vi "FPGA Target Approach RetractionA2copyAidanV2.vi"() -> ()   [LabVIEW 2012]
uses:
  <vilib>/rvi/FXPMathLib/basic elements/FxpIntAccumulator/subVIs/nifxpmath_IntAccumulator_SimConfig.ctl
  <vilib>/rvi/FXPMathLib/basic elements/FxpIntAccumulator/simVIs/DllFxpIntAccumulator_sub.vi
  <vilib>/rvi/Emulation/niFpgaSctlEmulationGetInTimedLoop.vi
  <vilib>/rvi/Emulation/niFpgaSctlEmulationGlobalWrite.vi
  <vilib>/rvi/eio/common/nirviEmuTemplateMethod_errors.vi
  <vilib>/rvi/interface/RandomDataEmulation/nirviRandomDataFPGAFIFO.vi
  <vilib>/rvi/interface/RandomDataEmulation/niFpgaRandomDataHandleErrors.vi
  <vilib>/rvi/FXPMathLib/basic elements/FxpIntAccumulator/XNode/nifxpmath_IntAccumulator.xnode
  <vilib>/eio/EIONode/EIONode.xnode
  <vilib>/rvi/Analysis/measure/butterworth/XNode/niFpgaButterworthFilter.xnode
  <vilib>/rvi/DataTransferAndStorage/Container/XNode/niFpgaContainer.xnode
  <vilib>/rvi/interface/RandomDataEmulation/nirviRandomDataFpgaReadWriteTemplate.vi
panel:
  in  "bounce distance control":i32
  in  "Set \"bounce\" distance or \nretract until":bool
  in  "Stop Fine Retraction\nand start next approach":bool
  out "Connector0/AI2":i16
  out "x*y":fxp<+/-,64,54>
  out "Numeric":i32
  out "initial setup complete":bool
  out "TF Phase":i16
  out "Approaches done and fully retracted":bool
  in  "Current Image":u8
  in  "Total Number of Images":u8
  out "Acoustic Sensor Signal":i16
  out "Step counter":i16
  out "fine indicator":i16
  in  "TF in Air":i32
  in  "Approach Minimum":i32
  in  "Approach Setpoint":i32
  in  "Fast Approach Offset":i32
  out "SummationfA":i32
  in  "Fine Approach Speed":fxp<+,64,38>
  out "SummationfR":i32
  in  "Fine Retraction Speed":fxp<+,64,38>
  out "SummationFA":i32
  out "Test Case Number Indicator":u8 format="%.1f"
  in  "Fast Approach Speed":fxp<+,64,38>
  in  "Approach":bool
  out "SummationFR":i32
  in  "Data Acquisition Rate":i16
  out "Ticks":i16
  out "Acoustic Sensor Phase":i16
  out "Tuning Fork Signal":i16
  in  "Fast Retraction Speed":fxp<+,64,38>
  out "Counter Indicator":fxp<+/-,64,32>
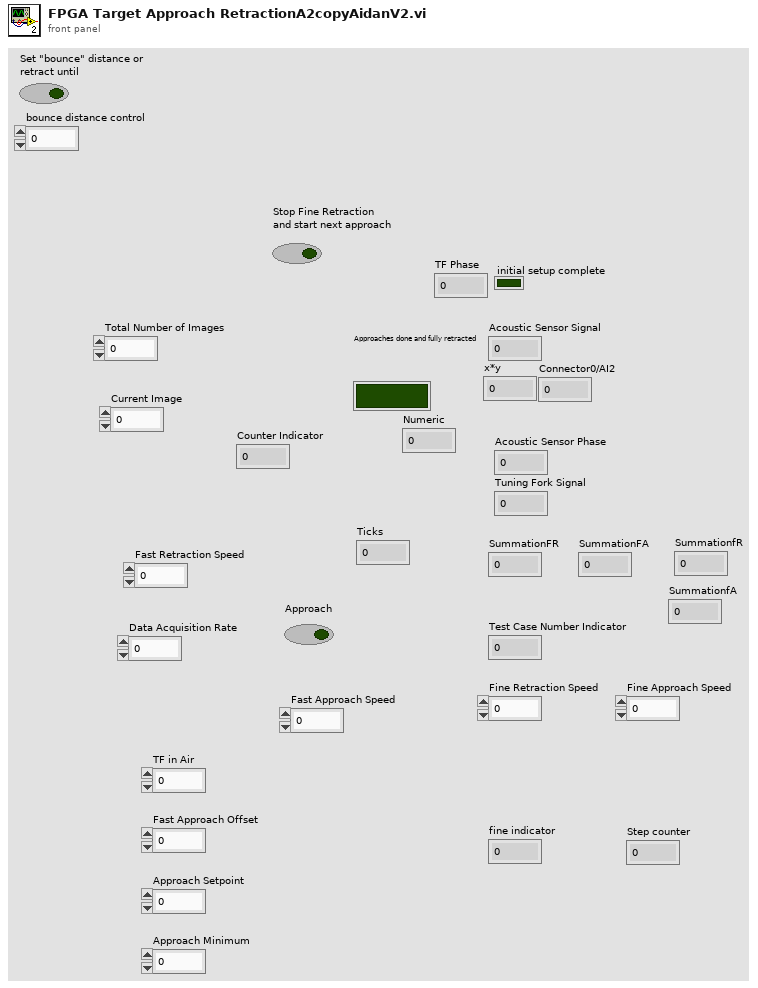
[diagram p1: front panel]
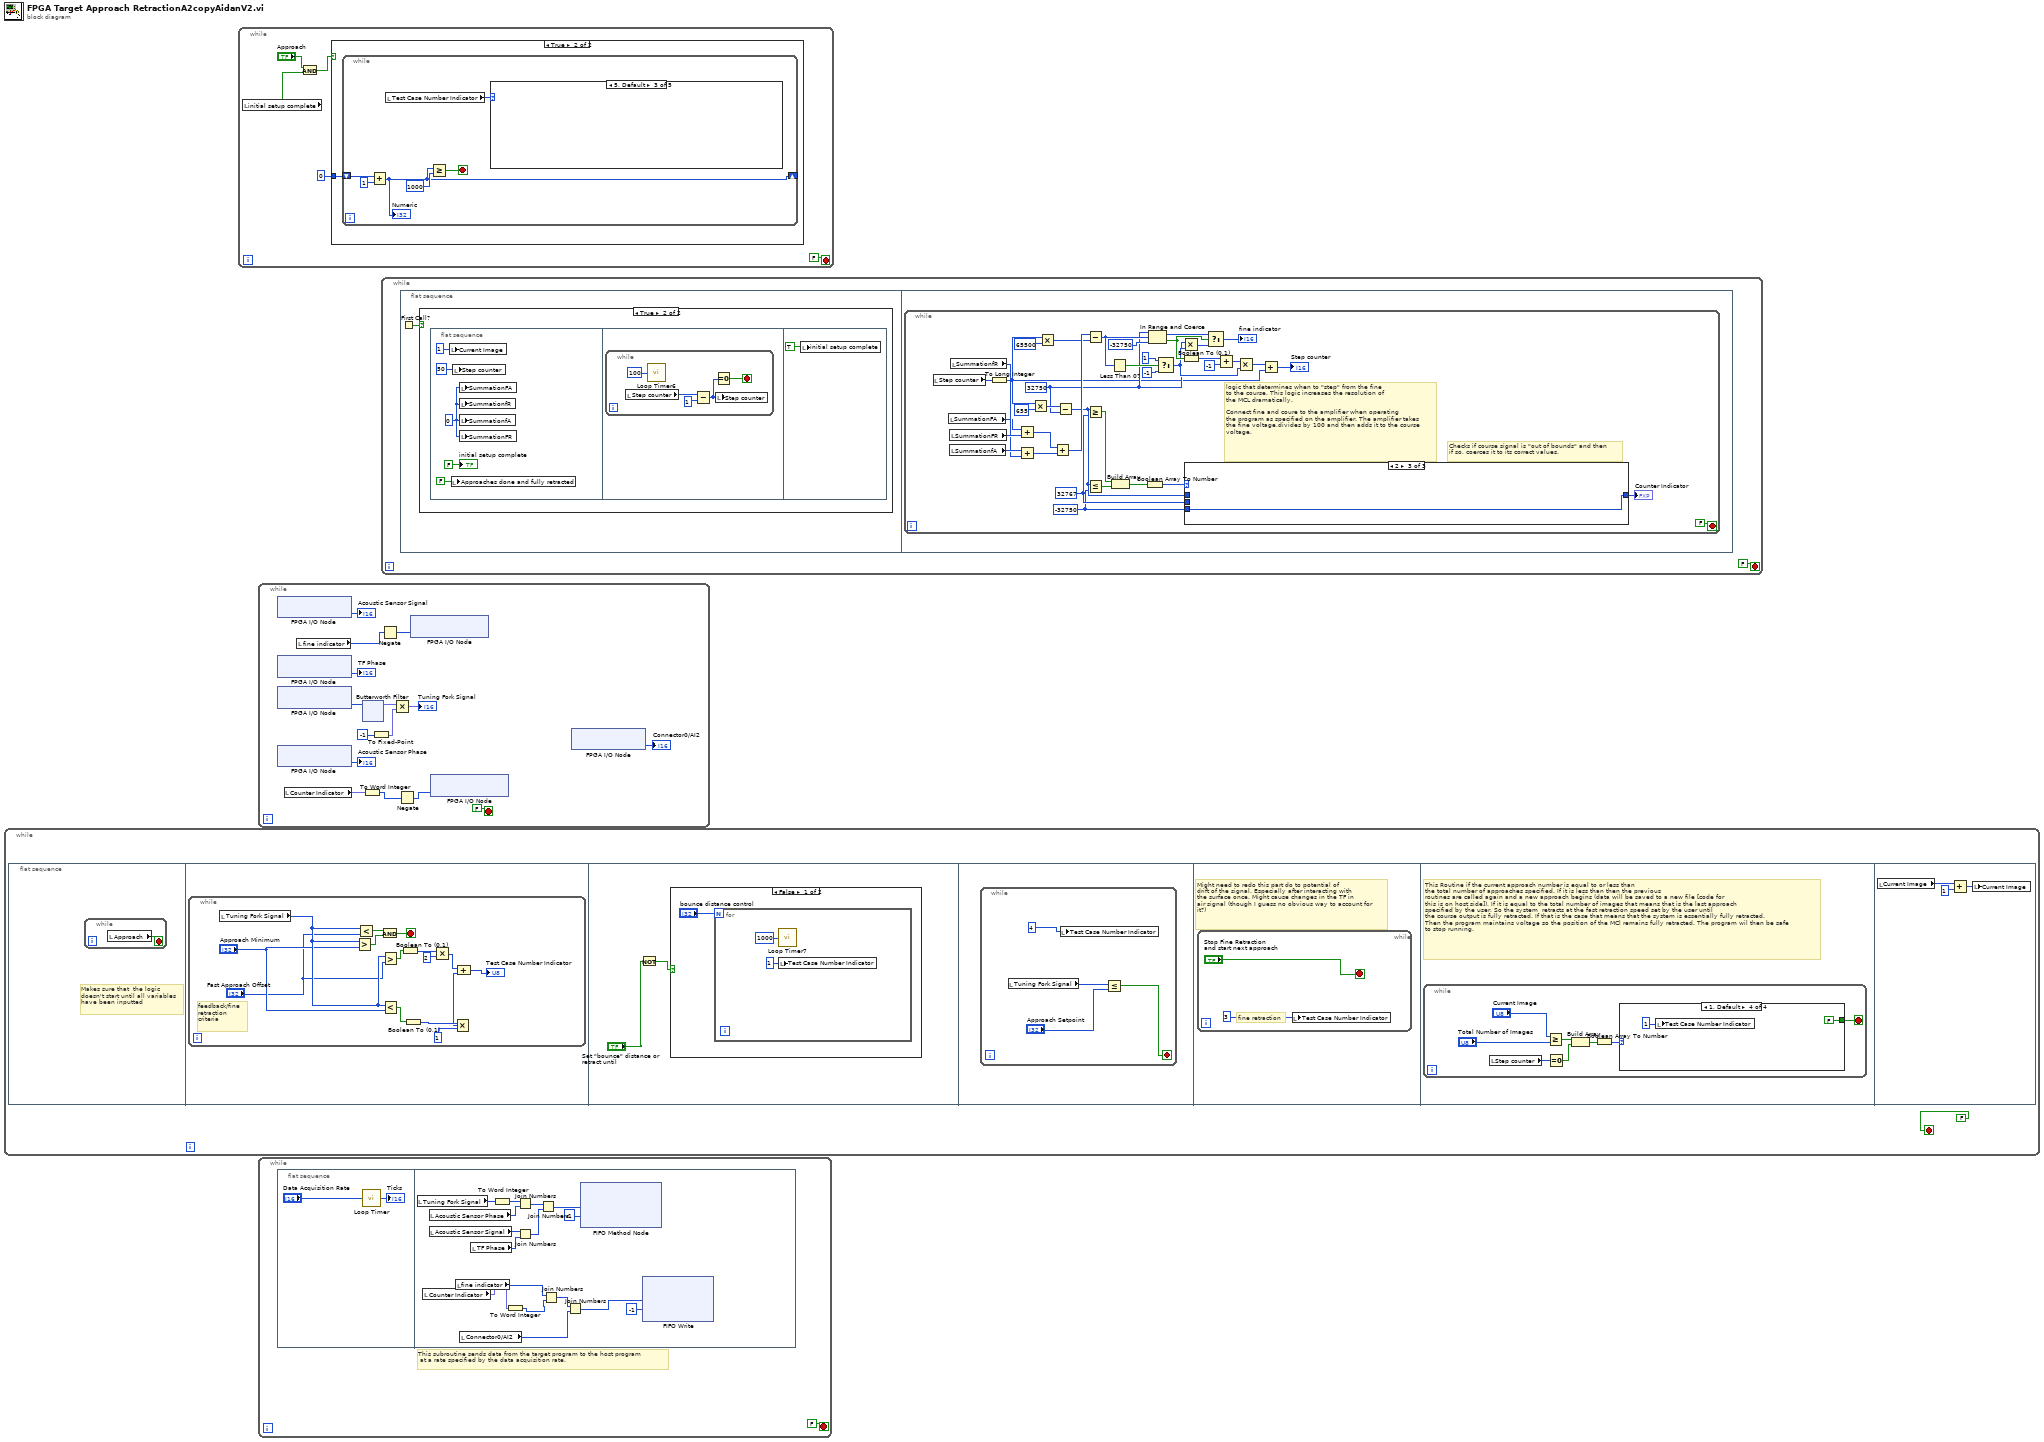
[diagram p0: block diagram]
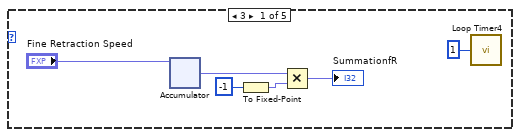
[diagram p3: hidden frame]
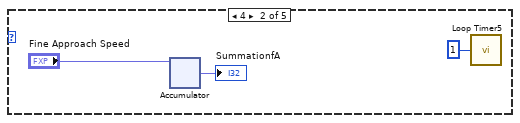
[diagram p4: hidden frame]
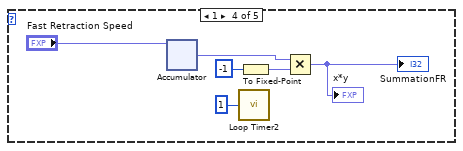
[diagram p5: hidden frame]
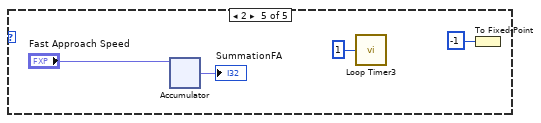
[diagram p6: hidden frame]
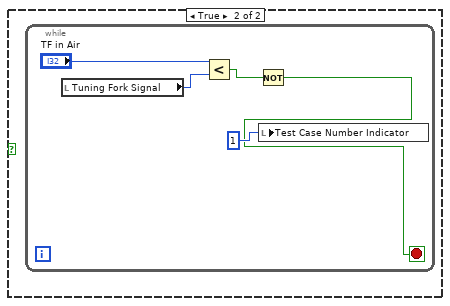
[diagram p10: hidden frame]
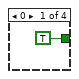
[diagram p11: hidden frame]
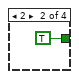
[diagram p12: hidden frame]
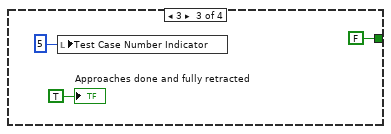
[diagram p13: hidden frame]
diagram:
  n1 = while {
    stop <- FALSE stop-if-true
    n2 = flat-sequence {
      frame #0 {
        # "Makes sure that  the logic  \ndoesn't start until all variables\nhave been inputted"
        n3 = while {
          stop <- w2 stop-if-true
          n4 = local read "Approach"() -> (w2:bool)
        }
      }
      frame #1 {
        n5 = while {
          stop <- w8 stop-if-true
          # "feedback/fine retraction criteria"
          n6 = local read "Tuning Fork Signal"() -> (w11:i16)
          n7 = Greater?(x=w11, y="Approach Minimum") -> (0:w9:bool)
          n8 = Less?(x=w11, y="Fast Approach Offset") -> (x < y?=w10:bool)
          n9 = And(x=w10, y=w9) -> (x .and. y?=w8:bool)
          n10 = Greater?(x=w11, y="Fast Approach Offset") -> (0:w17:bool)
          n11 = Less?(x=w11, y="Approach Minimum") -> (x < y?=w12:bool)
          n12 = Boolean To (0,1)(Boolean=w17) -> (0, 1=w16:i16)
          n13 = Boolean To (0,1)(Boolean=w12) -> (0, 1=w13:i16)
          n14 = Multiply(x=w16, y=i16 2) -> (x*y=w6:i16)
          n15 = Multiply(x=w13, y=i16 1) -> (x*y=w5:i16)
          n16 = Compound Arithmetic op=ADD(w6, w5) -> (→"Test Case Number Indicator":i16)
        }
      }
      frame #2 {
        n17 = Not(x="Set \"bounce\" distance or \nretract until") -> (.not. x?=w18:bool)
        n18 = case shown="False" w18 {
          frame False {
            n19 = for {
              N: "bounce distance control" -> [_]
              n20 = call "Loop Timer7"("Count(mSec)"=u32 1000) -> ()  [unwired: 1 out]
              n21 = local write "Test Case Number Indicator"(u8 1 ("Test Case Number Indicator")) -> ()
            }
          }
          frame True {
            n22 = while {
              stop <- w23 stop-if-true
              n23 = local read "Tuning Fork Signal"() -> (w25:i16)
              n24 = Less?(x="TF in Air", y=w25) -> (x < y?=w24:bool)
              n25 = Not(x=w24) -> (.not. x?=w23:bool)
              n26 = local write "Test Case Number Indicator"(i16 1) -> ()
            }
          }
        }
      }
      frame #3 {
        n27 = while {
          stop <- w28 stop-if-true
          n28 = local read "Tuning Fork Signal"() -> (w29:i16)
          n29 = local write "Test Case Number Indicator"(u8 4 ("Test Case Number Indicator")) -> ()
          n30 = Less Or Equal?(x=w29, y="Approach Setpoint") -> (x <= y?=w28:bool)
        }
      }
      frame #4 {
        # "Might need to redo this part do to potential of\ndrift of the signal. Especially after interacting with \nthe surface once. Might cause changes in the TF in \nair signal (though I guess no obvious way to account for\nit?)"
        n31 = while {
          stop <- "Stop Fine Retraction\nand start next approach" stop-if-true
          # "fine retraction"
          n32 = local write "Test Case Number Indicator"(i16 3) -> ()
        }
      }
      frame #5 {
        # "This Routine if the current approach number is equal to or less than \nthe total number of approaches specified. If it is less than then the previous \nroutines are called again and a new approach begins (data will be saved to a new file [code for \nthis is on host side]). If it is equal to the total number of images that means that is the last approach\nspecified by the user. So the system  retracts at the fast retraction speed set by the user until\nthe course output is fully retracted. If that is the case that means that the system is essentially fully retracted. \nThen the program maintains voltage so the position of the MCl remains fully retracted. The program wil then be safe\nto stop running."
        n33 = while {
          stop <- w34 stop-if-true
          n34 = local read "Step counter"() -> (w39:i16)
          n35 = Greater Or Equal?(x="Current Image", y="Total Number of Images") -> (x >= y?=w38:bool)
          n36 = Equal To 0?(x=w39) -> (x = 0?=w37:bool)
          n37 = Build Array(w38, w37) -> (w36:bool[])
          n38 = Boolean Array To Number(Boolean array=w36) -> (number=w35:u8)
          n39 = case shown="1, Default" w35 {
            tunnel: [TRUE TRUE FALSE FALSE] -> w34
            frame 0 {
            }
            frame 2 {
            }
            frame 3 {
              n40 = local write "Test Case Number Indicator"(i16 5 ("Test Case Number Indicator")) -> ()
              "Approaches done and fully retracted" <- TRUE ("Approaches done and fully retracted")
            }
            frame 1, Default {
              n41 = local write "Test Case Number Indicator"(i16 1) -> ()
            }
          }
        }
      }
      frame #6 {
        n42 = local read "Current Image"() -> (w50:u8)
        n43 = Add(x=w50, y=u8 1) -> (x+y=w49:u8)
        n44 = local write "Current Image"(w49) -> ()
      }
    }
  }
  n45 = while {
    stop <- FALSE stop-if-true
    n46 = local read "initial setup complete"() -> (w53:bool)
    n47 = And(x="Approach", y=w53) -> (x .and. y?=w52:bool)
    n48 = case shown="True" w52 {
      tunnel: i16 0 -> [_ w57]
      frame False {
      }
      frame True {
        n49 = while {
          shift-right: [w58] -> _
          shift-left: w57 -> [w61]
          stop <- w62 stop-if-true
          n50 = Add(x=w61, y=1) -> (x+y=w58:i32)
          "Numeric" <- w58
          n51 = local read "Test Case Number Indicator"() -> (w63:u8)
          n52 = Greater Or Equal?(x=w58, y=1000) -> (x >= y?=w62:bool)
          n53 = case shown="5, Default" w63 {
            frame 3 {
              n54 = xnode "Accumulator"("x"="Fine Retraction Speed") -> ("s"=w64:fxp<+,64,38>)  [unwired: 4 in, 1 out]
              n55 = To Fixed-Point(number=i16 -1) -> (fixed-point=w67:fxp<+/-,16,16>)  [unwired: 1 in]
              n56 = Multiply(x=w64, y=w67) -> (x*y=→"SummationfR":fxp<+/-,64,54>)
              n57 = call "Loop Timer4"("Count(uSec)"=i16 1) -> ()  [unwired: 1 out]
            }
            frame 4 {
              n58 = xnode "Accumulator"("x"="Fine Approach Speed") -> ("s"=→"SummationfA":fxp<+,64,38>)  [unwired: 4 in, 1 out]
              n59 = call "Loop Timer5"("Count(uSec)"=i16 1) -> ()  [unwired: 1 out]
            }
            frame 5, Default {
            }
            frame 1 {
              n60 = xnode "Accumulator"("x"="Fast Retraction Speed") -> ("s"=w130:fxp<+,64,38>)  [unwired: 4 in, 1 out]
              n61 = call "Loop Timer2"("Count(uSec)"=i16 1) -> ()  [unwired: 1 out]
              n62 = To Fixed-Point(number=i16 -1) -> (fixed-point=w128:fxp<+/-,16,16>)  [unwired: 1 in]
              n63 = Multiply(x=w130, y=w128) -> (x*y=→"SummationFR" →"x*y":fxp<+/-,64,54>)
            }
            frame 2 {
              n64 = xnode "Accumulator"("x"="Fast Approach Speed") -> ("s"=→"SummationFA":fxp<+,64,38>)  [unwired: 4 in, 1 out]
              n65 = call "Loop Timer3"("Count(uSec)"=i16 1) -> ()  [unwired: 1 out]
              n66 = To Fixed-Point(number=i16 -1) -> ()  [unwired: 1 in, 1 out]
            }
          }
        }
      }
    }
  }
  n67 = while {
    stop <- FALSE stop-if-true
    n68 = xnode "FPGA I/O Node"() -> ("Connector0/AI5"=→"Acoustic Sensor Signal":i16)  [unwired: 1 in, 1 out]
    n69 = xnode "FPGA I/O Node"() -> ("Connector0/AI4"=→"TF Phase":i16)  [unwired: 1 in, 1 out]
    n70 = xnode "FPGA I/O Node"() -> ("Connector0/AI7"=w200:i16)  [unwired: 1 in, 1 out]
    n71 = xnode "FPGA I/O Node"() -> ("Connector0/AI6"=→"Acoustic Sensor Phase":i16)  [unwired: 1 in, 1 out]
    n72 = local read "Counter Indicator"() -> (w197:fxp<+/-,64,32>)
    n73 = local read "fine indicator"() -> (w193:i16)
    n74 = xnode "Butterworth Filter"("input data"=w200) -> ("output data"=w204:fxp<+/-,20,20>)  [unwired: 2 in]
    n75 = To Word Integer(number=w197) -> (16bit integer=w195:i16)
    n76 = To Fixed-Point(number=i16 -1) -> (fixed-point=w203:fxp<+/-,16,16>)  [unwired: 1 in]
    n77 = Negate(x=w193) -> (-x=w192:i16)
    n78 = Multiply(x=w204, y=w203) -> (x*y=→"Tuning Fork Signal":fxp<+/-,36,36>)
    n79 = Negate(x=w195) -> (-x=w194:i16)
    n80 = xnode "FPGA I/O Node"("Connector0/AO6"=w192) -> ()  [unwired: 1 in, 1 out]
    n81 = xnode "FPGA I/O Node"("Connector0/AO7"=w194) -> ()  [unwired: 1 in, 1 out]
    n82 = xnode "FPGA I/O Node"() -> ("Connector0/AI2"=→"Connector0/AI2":i16)  [unwired: 1 in, 1 out]
  }
  n83 = while {
    stop <- FALSE stop-if-true
    # "This subroutine sends data from the target program to the host program\n at a rate specified by the data acquisition rate."
    n84 = flat-sequence {
      frame #0 {
        n85 = call "Loop Timer"("Count(uSec)"="Data Acquisition Rate") -> ("Tick Count(uSec)"=→"Ticks":u32)
      }
      frame #1 {
        n86 = local read "Tuning Fork Signal"() -> (w231:i16)
        n87 = local read "Counter Indicator"() -> (w222:fxp<+/-,64,32>)
        n88 = local read "Acoustic Sensor Phase"() -> (w229:i16)
        n89 = local read "Acoustic Sensor Signal"() -> (w225:i16)
        n90 = local read "fine indicator"() -> (w218:i16)
        n91 = local read "Connector0/AI2"() -> (w216:i16)
        n92 = local read "TF Phase"() -> (w224:i16)
        n93 = To Word Integer(number=w231) -> (16bit integer=w228:i16)
        n94 = To Word Integer(number=w222) -> (16bit integer=w219:i16)
        n95 = Join Numbers(hi=w228, lo=w229) -> ((hi.lo)=w227:u32)
        n96 = Join Numbers(hi=w225, lo=w224) -> ((hi.lo)=w223:u32)
        n97 = Join Numbers(hi=w227, lo=w223) -> ((hi.lo)=w230:u64)
        n98 = Join Numbers(hi=w218, lo=w219) -> ((hi.lo)=w217:u32)
        n99 = Join Numbers(hi=w217, lo=w216) -> ((hi.lo)=w221:u64)
        n100 = xnode ("FIFO Method Node")("Element"=w230, "Timeout"=i16 -1) -> ()  [unwired: 1 in, 2 out]
        n101 = xnode "FIFO Write"("Element"=w221, "Timeout"=-1) -> ()  [unwired: 1 in, 2 out]
      }
    }
  }
  n102 = while {
    stop <- FALSE stop-if-true
    n103 = flat-sequence {
      frame #0 {
        n104 = First Call?() -> (First Call?: T/F=w233:bool)
        n105 = case shown="True" w233 {
          frame False {
          }
          frame True {
            n106 = flat-sequence {
              frame #0 {
                w236 = i16 0
                n107 = local write "Current Image"(i16 1) -> ()
                n108 = local write "Approaches done and fully retracted"(FALSE ("Approaches done and fully retracted")) -> ()
                n109 = local write "Step counter"(i16 50) -> ()
                n110 = local write "SummationFA"(w236) -> ()
                n111 = local write "SummationfR"(w236) -> ()
                n112 = local write "SummationfA"(w236) -> ()
                n113 = local write "SummationFR"(w236) -> ()
                "initial setup complete" <- FALSE
              }
              frame #1 {
                n114 = while {
                  stop <- w239 stop-if-true
                  n115 = local read "Step counter"() -> (w242:i16)
                  n116 = call "Loop Timer6"("Count(mSec)"=u32 100) -> ()  [unwired: 1 out]
                  n117 = Subtract(x=w242, y=i16 1) -> (x-y=w240:i16)
                  n118 = Equal To 0?(x=w240) -> (x = 0?=w239:bool)
                  n119 = local write "Step counter"(w240) -> ()
                }
              }
              frame #2 {
                n120 = local write "initial setup complete"(TRUE) -> ()
              }
            }
          }
        }
      }
      frame #1 {
        n121 = while {
          stop <- FALSE stop-if-true
          w246 = i16 -32750
          w247 = i16 32767
          w256 = i16 32750
          # "Checks if course signal is \"out of bounds\" and then\nif so, coerces it to its correct values."
          # "logic that determines when to \"step\" from the fine\nto the course. This logic increases the resolution of\nthe MCL dramatically. \n\nConnect fine and coure to the amplifier when operating\nthe program as specified on the amplifier. The amplifier takes\nthe fine voltage,divides by 100 and then adds it to the course\nvoltage."
          n122 = local read "Step counter"() -> (w255:i16)
          n123 = local read "SummationFA"() -> (w258:i32)
          n124 = local read "SummationFR"() -> (w282:i32)
          n125 = local read "SummationfA"() -> (w260:i32)
          n126 = local read "SummationfR"() -> (w259:i32)
          n127 = To Long Integer(number=w255) -> (32bit integer=w254:i32)
          n128 = Add(x=w258, y=w282) -> (x+y=w281:i32)
          n129 = Add(x=w260, y=w259) -> (x+y=w280:i32)
          n130 = Multiply(x=w254, y=i16 655) -> (x*y=w257:i32)
          n131 = Multiply(x=w254, y=65500) -> (x*y=w277:i32)
          n132 = Add(x=w281, y=w280) -> (x+y=w279:i32)
          n133 = Subtract(x=w257, y=w256) -> (x-y=w248:i32)
          n134 = Subtract(x=w279, y=w277) -> (x-y=w274:i32)
          n135 = Greater Or Equal?(x=w248, y=w247) -> (x >= y?=w252:bool)
          n136 = Less Or Equal?(x=w248, y=w246) -> (x <= y?=w251:bool)
          n137 = Less Than 0?(x=w274) -> (x < 0?=w273:bool)
          n138 = Build Array(w252, w251) -> (w249:bool[])
          n139 = Boolean Array To Number(Boolean array=w249) -> (number=w250:u8)
          n140 = In Range and Coerce(upper limit=w256, x=w274, lower limit=i16 -32750) -> (coerced(x)=w276:i32, In Range?=w266:bool)
          n141 = Select(t=i16 1, s=w273, f=i16 -1) -> (s? t:f=w262:i16)
          n142 = Multiply(x=w256, y=w262) -> (x*y=w270:i16)
          n143 = Boolean To (0,1)(Boolean=w266) -> (0, 1=w265:i16)
          n144 = case shown="2" w250 {
            tunnel: [w283 w284 w285] -> w253
            tunnel: w248 -> [w283 _ _]
            tunnel: w247 -> [_ w284 _]
            tunnel: w246 -> [_ _ w285]
            frame 0, Default {
            }
            frame 1 {
            }
            frame 2 {
            }
          }
          "Counter Indicator" <- w253
          n145 = Select(t=w276, s=w266, f=w270) -> (s? t:f=→"fine indicator":i32)
          n146 = Add(x=w265, y=i16 -1) -> (x+y=w263:i16)
          n147 = Multiply(x=w263, y=w262) -> (x*y=w261:i16)
          n148 = Add(x=w261, y=w254) -> (x+y=→"Step counter":i32)
        }
      }
    }
  }
